vi "crh_backup.vi"() -> ()   [LabVIEW 2012]
panel:
  out "error out 2":errorcluster
  out "OK 2":bool
  out "OK":bool
  out "folder 2":string
  out "concatenated string 2":string
  out "concatenated string":string
  in  "folder":string="QAMT01\\CRH3605"
  out "error out":errorcluster
  in  "error in (no error)":errorcluster
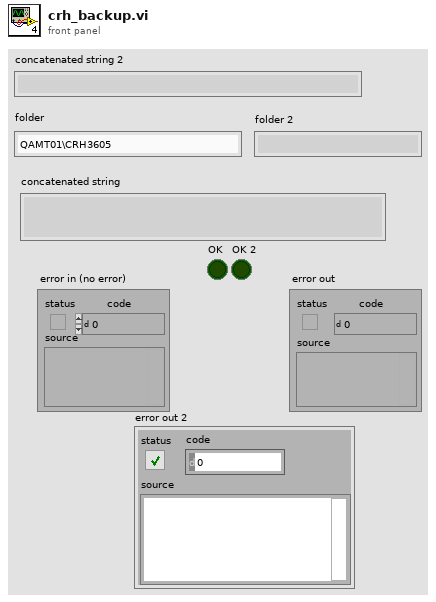
[diagram p1: front panel]
types:
  T1 = enum16{"open", "replace", "create", "open or create", "replace or create", "replace or create with confirmation"}
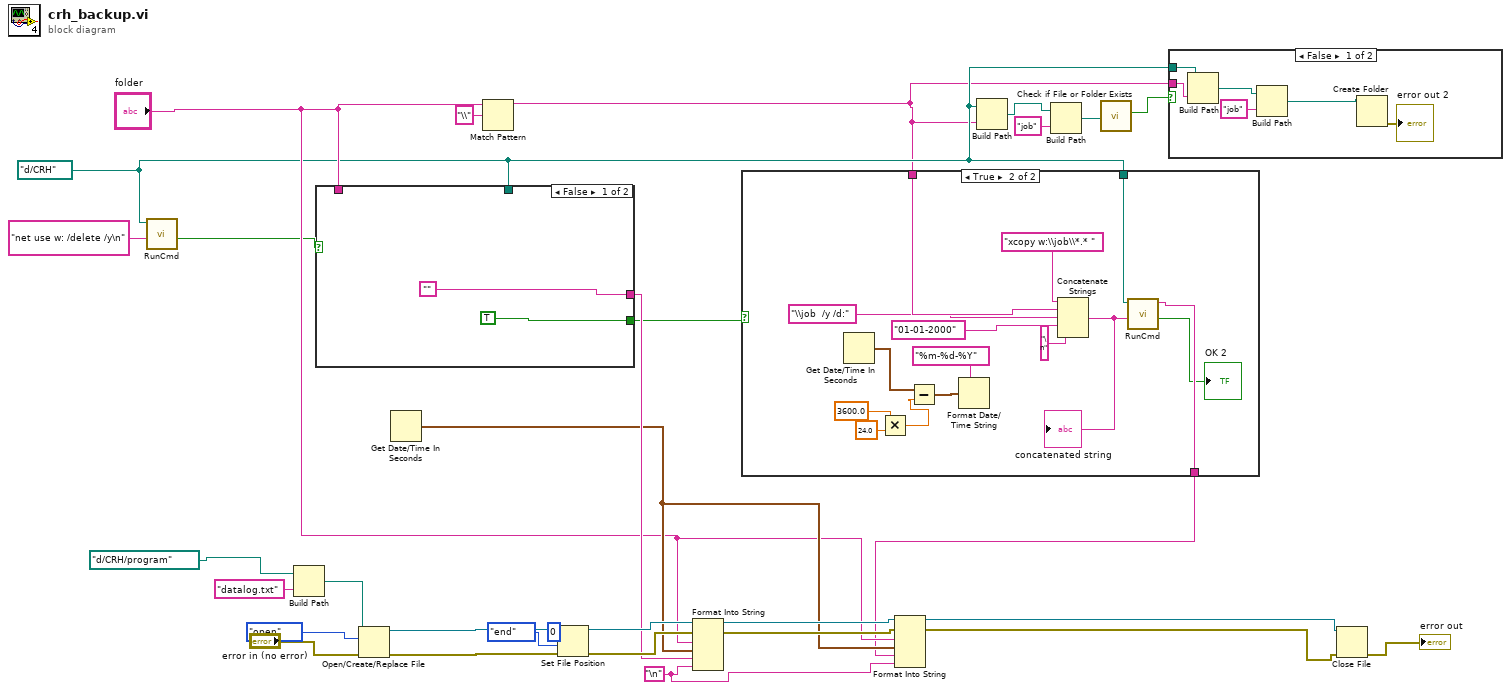
[diagram p0: block diagram]
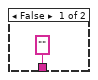
[diagram p3: hidden frame]
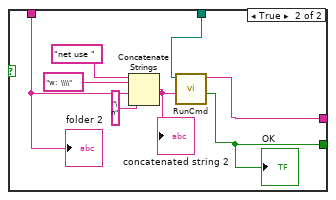
[diagram p4: hidden frame]
diagram:
  w8 = "\n"
  w7 = path "d:/CRH" ("working directory")
  n1 = call "RunCmd.vi"("Cmd String"="net use w: /delete /y\n" ("string"), "working directory"=w7) -> ("OK"=w1:bool)  [unwired: 8 in, 1 out]
  n2 = Build Path(base path=path "d:/CRH/program", name or relative path="datalog.txt") -> (appended path=w23:path)
  n3 = case shown="False" w1 {
    tunnel: [TRUE w35] -> w16
    tunnel: ["" w36] -> w19
    tunnel: "folder" -> [_ w38]
    tunnel: w7 -> [_ w37]
    frame False {
    }
    frame True {
      n4 = Concatenate Strings("net use " ("string"), "w:  \\\\" ("string"), w38, "\n" ("string")) -> (w41:string)
      "concatenated string 2" <- w41
      n5 = call "RunCmd.vi"("Cmd String"=w41, "working directory"=w37) -> ("OK"=w35:bool, "Output"=w36:string)  [unwired: 8 in]
      "OK" <- w35
      "folder 2" <- w38
    }
  }
  n6 = Open/Create/Replace File(file path (use dialog)=w23, error in="error in (no error)", operation (0:open)=T1."open") -> (refnum out=w28:refnum<file>, error out=w27:errorcluster)  [unwired: 3 in, 1 out]
  n7 = Get Date/Time In Seconds() -> (seconds since 1Jan1904=w11:timestamp)
  n8 = Match Pattern(string="folder", regular expression="\\") -> (before substring=w6:string)  [unwired: 1 in, 3 out]
  n9 = Set File Position(offset (in bytes) (0)=i64 0, refnum=w28, from (0:start)=enum16{"start", "end", "current"}."end", error in=w27) -> (refnum out=w21:refnum<file>, error out=w20:errorcluster)
  n10 = Format Into String(initial string=w21, error in=w20, "folder", w11, w19, w8) -> (resulting string=w12:refnum<file>, error out=w14:errorcluster)  [unwired: 1 in]
  n11 = case shown="True" w16 {
    tunnel: w6 -> [_ w57]
    tunnel: w7 -> [_ w48]
    tunnel: ["" ("Output") w46] -> w9
    frame False {
    }
    frame True {
      n12 = Get Date/Time In Seconds() -> (seconds since 1Jan1904=w50:timestamp)
      n13 = Multiply(x=3600.0, y=24.0) -> (x*y=w52:dbl)
      n14 = Subtract(x=w50, y=w52) -> (x-y=w53:timestamp)
      n15 = Format Date/Time String(time format string (%c)="%m-%d-%Y", seconds (now)=w53) -> ()  [unwired: 1 in, 1 out]
      n16 = Concatenate Strings("xcopy w:\\job\\*.* " ("string"), w57, "\\job  /y /d:" ("string"), "01-01-2000" ("string"), "\n" ("string")) -> (w47:string)
      "concatenated string" <- w47
      n17 = call "RunCmd.vi"("Cmd String"=w47, "working directory"=w48) -> ("OK"=→"OK 2":bool, "Output"=w46:string)  [unwired: 8 in]
    }
  }
  n18 = Format Into String(initial string=w12, error in=w14, "folder", w11, w9, w8) -> (resulting string=w15:refnum<file>, error out=w13:errorcluster)  [unwired: 1 in]
  n19 = Build Path(base path=w7, name or relative path=w6) -> (appended path=w4:path)
  n20 = Build Path(base path=w4, name or relative path="job") -> (appended path=w3:path)
  n21 = call <vilib>:"Check if File or Folder Exists.vi"("path"=w3) -> ("file or folder exists?"=w2:bool)  [unwired: 8 in, 2 out]
  n22 = case shown="False" w2 {
    tunnel: w7 -> [w62 _]
    tunnel: w6 -> [w61 _]
    frame False {
      n23 = Build Path(base path=w62, name or relative path=w61) -> (appended path=w60:path)
      n24 = Build Path(base path=w60, name or relative path="job") -> (appended path=w58:path)
      n25 = Create Folder(path (use dialog)=w58) -> (error out=→"error out 2":errorcluster)  [unwired: 2 in, 2 out]
    }
    frame True {
    }
  }
  n26 = Close File(refnum=w15, error in=w13) -> (error out=→"error out":errorcluster)  [unwired: 1 out]
